vi "Write Recombination Rate.vi"(8 "error in (no error)":errorcluster, 10 "Recombination Rate":dbl, 11 "GA Core in":refnum<class "GA Core.lvclass">) -> (0 "error out":errorcluster, 3 "GA Core out":refnum<class "GA Core.lvclass">)   [LabVIEW 2016, in "GA Core.lvclass"]
uses:
  GA Core.lvclass
  GA Core.lvclass/GA Core.ctl
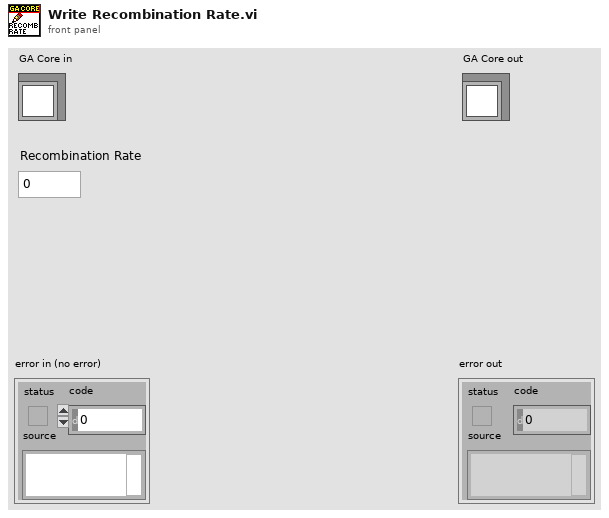
[diagram p1: front panel]
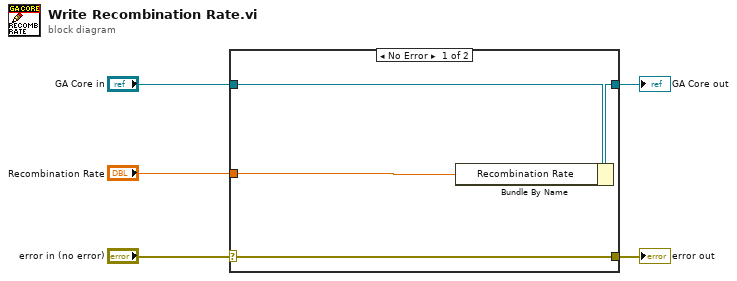
[diagram p0: block diagram]
diagram:
  n1 = case shown="No Error" "error in (no error)" {
    selector: "error in (no error)" -> [w9 w10]
    tunnel: [w9 w10] -> w4
    tunnel: [w7 w11] -> w2
    tunnel: "GA Core in" -> [w8 w11]
    tunnel: "Recombination Rate" -> [w6 _]
    frame No Error {
      n2 = Bundle By Name(cluster=w8, "Recombination Rate"=w6) -> (w7:refnum<class "GA Core.lvclass">)
    }
    frame Error {
    }
  }
  "error out" <- w4
  "GA Core out" <- w2
